vi "acquire_trace.vi"() -> ()   [LabVIEW 2015, in "oscilloscope.lvlib"]
doc: "This example shows how to use autosetup and acquire a waveform on a single channel for acquiring waveforms in a loop until stopped by user."
uses:
  oscilloscope.lvlib
  osc_channel.ctl
  osc_stats.ctl
  simulate_trace.ctl
  Global.vi
  oskar_tools/oskar_tools.lvlib
panel:
  out "SQUID":string="3"
  in  "stop":bool
  in  "Tab Control":T1(tab)
  out "Saving":bool
  out "Waveform Data":waveform(dbl)[](graph)=[{"t0"=timestamp(0 s since 1904-01-01), "dt"=9.999999999999999e-10, "Y"=array[700 elements]}, {"t0"=timestamp(0 s since 1904-01-01), "dt"=9.999999999999999e-10, "Y"=array[700 elements]}]
  in  "Points":i32=700
  out "dt":dbl=9.999999999999999e-10 format="%#_2e"
  out "Repeat":u32=19
  out "Scope":cluster{"Manufacturer":string, "Model":string}={"Manufacturer"="Skynet", "Model"="T1000"}
  in  "record stats.":bool[](array[boolean])=[TRUE, TRUE]
  out "Statistics":T2[](array[typedef])=[{"min"=1.6569042028773572e-05, "t_min"=6.999999999999999e-09, "max"=1.0011047855736102, "t_max"=9.999999999999998e-08, "range"=1.0010882165315813, "mean"=0.07129498123141252, "stdev"=0.15325605925926297}, {"min"=3.275572243336018e-05, "t_min"=5.999999999999999e-09, "max"=0.25, "t_max"=8.399999999999998e-08, "range"=0.24996724427756664, "mean"=0.048822392356695436, "stdev"=0.06410639456034639}]
  in  "noise":dbl[](array[numeric])=[0.005, 0.002] format="%#_13g"
  in  "Channels":T3[](array[typedef])=[{"channel name"="CHANNEL1", "probe attenuation"=1.0, "vertical offset"=0.0, "vertical range"=10.0, "vertical coupling"=1, "input impedance"=50.0}, {"channel name"="CHANNEL2", "probe attenuation"=1.0, "vertical offset"=0.0, "vertical range"=0.5, "vertical coupling"=1, "input impedance"=50.0}] caption="Settings" {"input impedance" format="%#_13g"; "vertical coupling" items=["AC", "DC", "GND"]; "vertical range" format="%.3f"; "vertical offset" format="%.3f"; "probe attenuation" format="%.3f"}
  in  "wait (ms)":u32=500
  in  "Bin size":i16=1
  in  "sample":dbl=7e-07
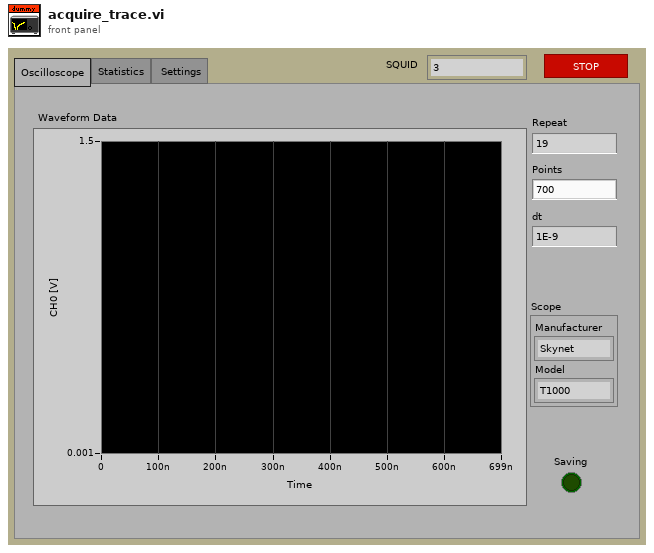
[diagram p1: front panel]
types:
  T1 = enum32{"Oscilloscope", "Statistics", " Settings"}
  T2 = typedef "oscilloscope.lvlib/osc_stats.ctl" = cluster{"min":dbl, "t_min":dbl, "max":dbl, "t_max":dbl, "range":dbl, "mean":dbl, "stdev":dbl}
  T3 = typedef "oscilloscope.lvlib/osc_channel.ctl" = cluster{"channel name":string, "probe attenuation":dbl, "vertical offset":dbl, "vertical range":dbl, "vertical coupling":i32, "input impedance":dbl}
  T4 = typedef "oscilloscope.lvlib/simulate_trace.ctl" = cluster{"N":i32, "x0":dbl, "dx":dbl, "noise":dbl, "A":dbl, "eff":dbl, "sigma":dbl, "tau":dbl}
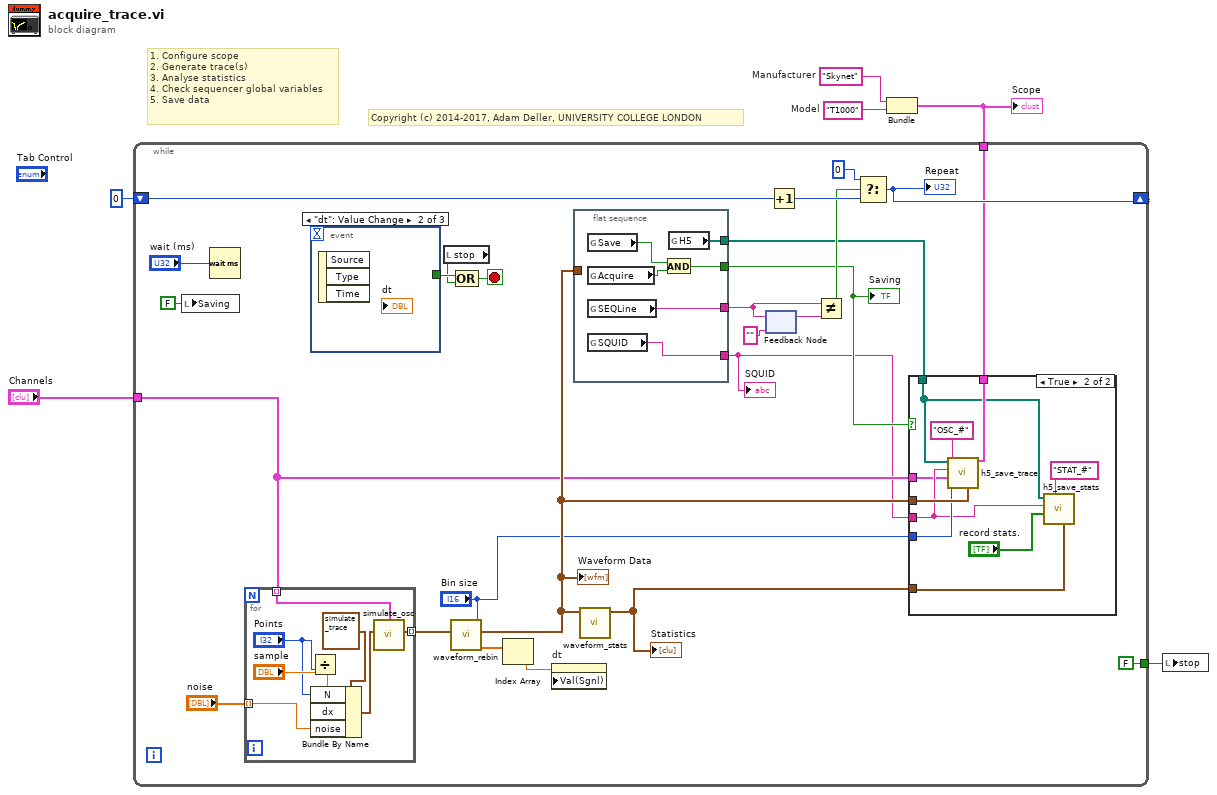
[diagram p0: block diagram]
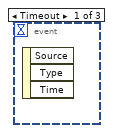
[diagram p3: hidden frame]
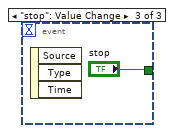
[diagram p4: hidden frame]
diagram:
  w2 = "T1000"  # Model
  w1 = "Skynet"  # Manufacturer
  # "Copyright (c) 2014-2017, Adam Deller, UNIVERSITY COLLEGE LONDON"
  # "1. Configure scope\n2. Generate trace(s)\n3. Analyse statistics\n4. Check sequencer global variables\n5. Save data"
  n1 = Bundle("Manufacturer"=w1, "Model"=w2) -> (w3:cluster{"Manufacturer":string, "Model":string})  [unwired: 1 in]
  "Scope" <- w3
  n2 = while {
    shift-right: [w29] -> _
    shift-left: u32 0 ("millisecond multiple") -> [w30]
    tunnel: [FALSE ("stop")] -> w5
    tunnel: "Channels" -> [w20]
    tunnel: w3 -> [w12]
    stop <- w31 stop-if-true
    n3 = local write "Saving"(FALSE ("Saving")) -> ()
    n4 = Wait (ms)(milliseconds to wait="wait (ms)") -> ()  [unwired: 1 out]
    n5 = for {
      tunnel: [w56] -> w23 mode=indexing
      tunnel: w20 -> [w57] mode=indexing
      tunnel: "noise" -> [w53] mode=indexing
      n6 = Divide(x="sample", y="Points") -> (x/y=w52:dbl)
      n7 = Bundle By Name(cluster=T4 {"N"=600, "x0"=-1e-07, "dx"=1e-09, "noise"=0.1, "A"=1.0, "eff"=0.25, "sigma"=1e-08, "tau"=1.42e-07} ("trace"), "N"="Points", "dx"=w52, "noise"=w53) -> (w51:T4)
      n8 = call "simulate_osc.vi"("CHAN"=w57, "trace"=w51) -> ("output waveform"=w56:waveform(dbl))  [unwired: 9 in]
    }
    n9 = event shown="[1] \"dt\": Value Change" {
      selector: _ -> [_ _ _]
      dyn-events: _ -> [_ _ _]
      timeout: _ -> [_ _ _]
      tunnel: [_ _ "stop"] -> w27
      event Timeout {
        n10 = event-data() -> ()  [unwired: 1 in, 3 out]
      }
      event "dt": Value Change {
        n11 = event-data() -> ()  [unwired: 1 in, 3 out]
      }
      event "stop": Value Change {
        n12 = event-data() -> ()  [unwired: 1 in, 3 out]
      }
    }
    n13 = local read "stop"() -> (w26:bool)
    n14 = call "waveform_rebin.vi"("Bin size"="Bin size", "Waveform Data IN"=w23) -> ("dt"=w22:dbl[], "Waveform Data OUT"=w24:waveform(dbl)[])  [unwired: 6 in, 1 out]
    "Waveform Data" <- w24
    n15 = Compound Arithmetic op=OR(w27, w26) -> (w31:bool)
    n16 = Index Array(array=w22) -> (element=w11:dbl)  [unwired: 1 in]
    n17 = property on="dt" class="DigNum (strict)"("Val(Sgnl)"=w11) -> ()  [unwired: 2 in, 2 out]
    n18 = flat-sequence {
      tunnel: w24 -> [_]
      tunnel: [w36] -> w15
      tunnel: [w35] -> w9
      tunnel: [w33] -> w8
      tunnel: [w34] -> w13
      frame #0 {
        n19 = global read "Global.vi" "Save"() -> (w37:bool)
        n20 = global read "Global.vi" "Acquire"() -> (w38:bool)
        n21 = global read "Global.vi" "SEQLine"() -> (w35:string)
        n22 = global read "Global.vi" "SQUID"() -> (w33:string)
        n23 = And(x=w37, y=w38) -> (x .and. y?=w36:bool)
        n24 = global read "Global.vi" "H5"() -> (w34:path[])
      }
    }
    n25 = call "waveform_stats.vi"("Waveform Data"=w24) -> ("stats"=w14:T2[])  [unwired: 7 in]
    "Statistics" <- w14
    n26 = feedback #1("" ("Seq")) -> (w10:string)
    n27 = feedback-in #1(w9) -> ()
    n28 = Increment(x=w30) -> (x+1=w18:u32)
    n29 = Not Equal?(x=w9, y=w10) -> (x != y?=w17:bool)
    n30 = Select(t=u32 0, s=w17, f=w18) -> (s? t:f=w29:u32)
    "Repeat" <- w29
    n31 = case shown="True" w15 {
      tunnel: w24 -> [_ w48]
      tunnel: w20 -> [_ w39]
      tunnel: w8 -> [_ w44]
      tunnel: "Bin size" -> [_ w45]
      tunnel: w14 -> [_ w40]
      tunnel: w13 -> [_ w43]
      tunnel: w12 -> [_ w46]
      frame False {
      }
      frame True {
        n32 = call "h5_save_trace.vi"("Waveform Data"=w48, "Scope"=w46, "TYPE"="OSC_#", "Bin size"=w45, "Settings"=w39, "SQUID"=w44, "H5"=w43) -> ()  [unwired: 4 in, 1 out]
        n33 = call "h5_save_stats.vi"("stats"=w40, "TYPE"="STAT_#", "record stats."="record stats.", "SQUID"=w44, "H5"=w43) -> ()  [unwired: 6 in, 1 out]
      }
    }
    "Saving" <- w15
    "SQUID" <- w8
  }
  n34 = local write "stop"(w5) -> ()
